vi "WPI_CameraParse URL.vi"(10 "Full":bool, 11 "URL":string="http://roborio-419-frc.local:1181/video?name=Camera&resolution=640x480&compression=40&fps=15") -> (0 "cgi string":string, 1 "parameters":T1(array[cluster]), 2 "port":i32, 3 "address":string)   [LabVIEW 2017]
panel:
  # "http://roboRIO-419-FRC.local:5800/?action=stream"
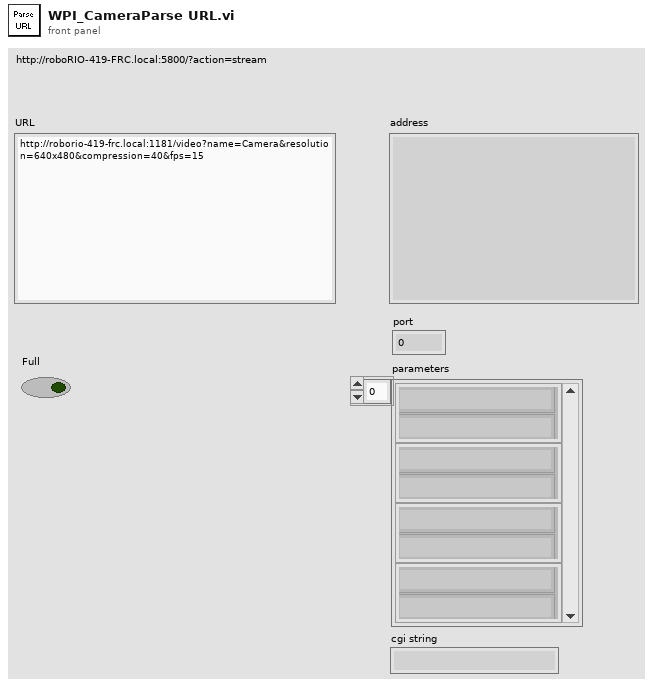
[diagram p1: front panel]
types:
  T1 = cluster{"token string":string, "token string 2":string}[]
  T2 = cluster{"token string":string, "offset past token":i32}
  T3 = cluster{"token string":string, "offset past token":i32}[]
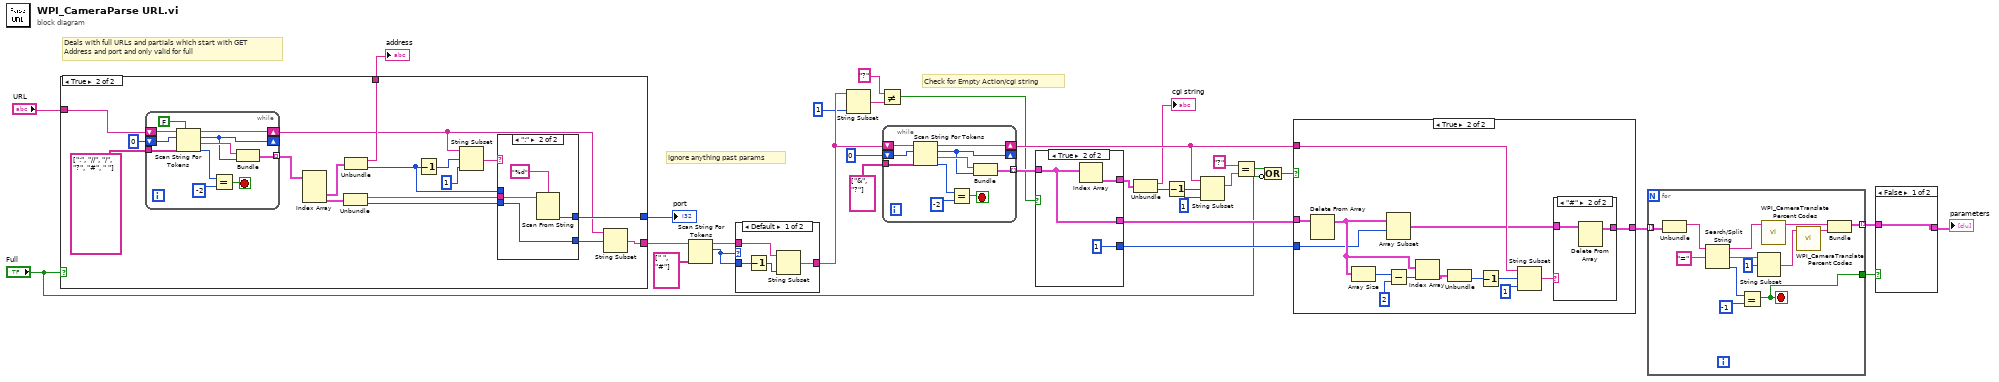
[diagram p0: block diagram]
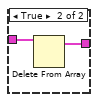
[diagram p4: hidden frame]
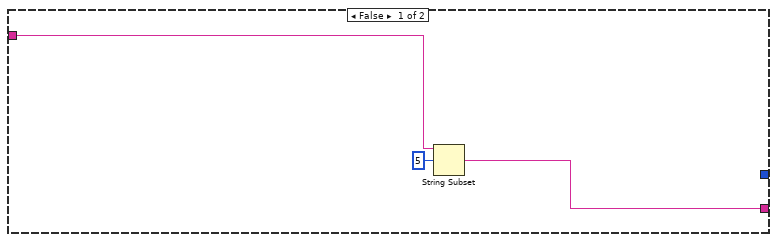
[diagram p5: hidden frame]
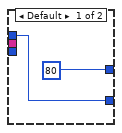
[diagram p6: hidden frame]
diagram:
  # "Check for Empty Action/cgi string"
  # "Ignore anything past params"
  # "Deals with full URLs and partials which start with GET \nAddress and port and only valid for full"
  n1 = case shown="True" "Full" {
    tunnel: [_ w47] -> w32
    tunnel: [_ w46] -> w31
    tunnel: "URL" -> [w35 w42]
    tunnel: [w34 w41] -> w12
    frame False {
      n2 = String Subset(string=w35, offset (0)=5) -> (substring=w34:string)  [unwired: 1 in]
    }
    frame True {
      n3 = while {
        tunnel: string[] [":", "//", "/", "?", "#", " "] -> [w69]
        shift-right: [w67] -> w43
        shift-left: w42 -> [w68]
        shift-right: [w60] -> _
        shift-left: 0 ("offset past token") -> [w66]
        tunnel: [w61] -> w50 mode=indexing
        stop <- w64 stop-if-true
        n4 = Scan String For Tokens(5:FALSE ("allow empty tokens? (F)"), 6:w69, 8:w66, 9:w68) -> (0:w62:i32, 1:w63:string, 2:w60:i32, 3:w67:string)  [unwired: 2 in]
        n5 = Equal?(x=w62, y=-2) -> (x = y?=w64:bool)
        n6 = Bundle("token string"=w63, "offset past token"=w60) -> (w61:T2)  [unwired: 1 in]
      }
      n7 = Index Array(array=w50) -> (element #2=w49:T2, element #3=w48:T2)  [unwired: 3 in, 1 out]
      n8 = Unbundle(w48) -> ("token string"=w40:string, "offset past token"=w45:i32)
      n9 = Unbundle(w49) -> ("token string"=w46:string, "offset past token"=w44:i32)
      n10 = Decrement(x=w44) -> (x-1=w38:i32)
      n11 = String Subset(string=w43, offset (0)=w38, length (rest)=1) -> (substring=w37:string)
      n12 = case shown="\":\"" w37 {
        tunnel: w40 -> [_ w58]
        tunnel: [80 w56] -> w47
        tunnel: w45 -> [_ w55]
        tunnel: [w53 w55] -> w36
        tunnel: w44 -> [w53 _]
        frame Default {
        }
        frame ":" {
          n13 = Scan From String(format string="%d", input string=w58) -> (output 1=w56:i32)  [unwired: 3 in, 3 out]
        }
      }
      n14 = String Subset(string=w43, offset (0)=w36) -> (substring=w41:string)  [unwired: 1 in]
    }
  }
  "address" <- w31
  "port" <- w32
  n15 = Scan String For Tokens(6:string[] [" ", "#"], 9:w12) -> (2:w9:i32, 3:w10:string)  [unwired: 4 in, 2 out]
  n16 = case shown="Default" w9 {
    tunnel: w9 -> [w71 _]
    tunnel: [w72 w74] -> w8
    tunnel: w10 -> [w73 w74]
    frame Default {
      n17 = Decrement(x=w71) -> (x-1=w70:i32)
      n18 = String Subset(string=w73, length (rest)=w70) -> (substring=w72:string)  [unwired: 1 in]
    }
    frame -2, -1 {
    }
  }
  n19 = String Subset(string=w8, length (rest)=1 ("length (rest)")) -> (substring=w6:string)  [unwired: 1 in]
  n20 = Not Equal?(x="?" ("format string"), y=w6) -> (x != y?=w3:bool)
  n21 = while {
    tunnel: string[] ["&", "?"] -> [w84]
    shift-right: [w82] -> w24
    shift-left: w8 -> [w83]
    shift-right: [w75] -> _
    shift-left: 0 ("offset past token") -> [w81]
    tunnel: [w76] -> w25 mode=indexing
    stop <- w79 stop-if-true
    n22 = Scan String For Tokens(6:w84, 8:w81, 9:w83) -> (0:w77:i32, 1:w78:string, 2:w75:i32, 3:w82:string)  [unwired: 3 in]
    n23 = Equal?(x=w77, y=-2) -> (x = y?=w79:bool)
    n24 = Bundle("token string"=w78, "offset past token"=w75) -> (w76:T2)  [unwired: 1 in]
  }
  n25 = case shown="True" w3 {
    tunnel: w25 -> [w85 w87]
    tunnel: [_ w88] -> w22
    tunnel: [w85 w87] -> w4
    tunnel: [_ 1] -> w2
    frame False {
    }
    frame True {
      n26 = Index Array(array=w87) -> (element=w88:T2)  [unwired: 1 in]
    }
  }
  n27 = Unbundle(w22) -> ("token string"=→"cgi string":string, "offset past token"=w28:i32)
  n28 = Decrement(x=w28) -> (x-1=w27:i32)
  n29 = String Subset(string=w24, offset (0)=w27, length (rest)=1) -> (substring=w19:string)
  n30 = Equal?(x="?" ("format string"), y=w19) -> (x = y?=w18:bool)
  n31 = Compound Arithmetic op=OR(w18, invert "Full") -> (w17:bool)
  n32 = case shown="True" w17 {
    tunnel: w4 -> [_ w93]
    tunnel: w24 -> [_ w97]
    tunnel: [_ w94] -> w23
    tunnel: w2 -> [_ w89]
    frame False {
    }
    frame True {
      n33 = Delete From Array(array=w93) -> (array with subset deleted=w92:T3)  [unwired: 2 in, 1 out]
      n34 = Array Size(array=w92) -> (size(s)=w91:i32)
      n35 = Array Subset(array=w92, index=w89) -> (w95:T3)  [unwired: 1 in]
      n36 = Subtract(x=w91, y=2) -> (x-y=w102:i32)
      n37 = Index Array(array=w92, index=w102) -> (element=w100:T2)
      n38 = Unbundle(w100) -> ("offset past token"=w101:i32)  [unwired: 1 out]
      n39 = Decrement(x=w101) -> (x-1=w98:i32)
      n40 = String Subset(string=w97, offset (0)=w98, length (rest)=1) -> (substring=w96:string)
      n41 = case shown="\"#\"" w96 {
        tunnel: w95 -> [w103 w105]
        tunnel: [w103 w104] -> w94
        frame "False", Default {
        }
        frame "#" {
          n42 = Delete From Array(array=w105) -> (array with subset deleted=w104:T3)  [unwired: 2 in, 1 out]
        }
      }
    }
  }
  n43 = for {
    tunnel: w23 -> [w118] mode=indexing
    tunnel: [w113] -> w14 mode=indexing
    tunnel: [w110] -> w15
    stop <- w110 stop-if-true
    n44 = Unbundle(w118) -> ("token string"=w114:string)  [unwired: 1 out]
    n45 = Search/Split String(string=w114, search string/char (-)="=" ("format string")) -> (substring before match=w109:string, match + rest of string=w116:string, offset of match=w111:i32)  [unwired: 1 in]
    n46 = Equal?(x=w111, y=-1 ("offset (0)")) -> (x = y?=w110:bool)
    n47 = String Subset(string=w116, offset (0)=1) -> (substring=w106:string)  [unwired: 1 in]
    n48 = call <vilib>:"WPI_CameraTranslate Percent Codes.vi"("String"=w109) -> ("String 2"=w108:string)  [unwired: 10 in]
    n49 = call <vilib>:"WPI_CameraTranslate Percent Codes.vi"("String"=w106) -> ("String 2"=w107:string)  [unwired: 10 in]
    n50 = Bundle("String 2"=w108, "String 2"=w107) -> (w113:cluster{"String 2":string, "String 2":string})  [unwired: 1 in]
  }
  n51 = case shown="False" w15 {
    tunnel: w14 -> [w119 w121]
    tunnel: [w119 w120] -> w13
    frame False {
    }
    frame True {
      n52 = Delete From Array(array=w121) -> (array with subset deleted=w120:cluster{"String 2":string, "String 2":string}[])  [unwired: 2 in, 1 out]
    }
  }
  "parameters" <- w13
